vi "Calculate_Velocity.vi"(2 "Times":T1 {"Accel fractional distance" format="%.2f"; "Accel time" format="%.7f"; "Total travel time" format="%.7f"}, 5 "Revs to travel":dbl format="%.2f") -> (0 "Acceleration":dbl format="%.2f", 1 "Max Velocity":dbl format="%.2f")   [LabVIEW 2018]
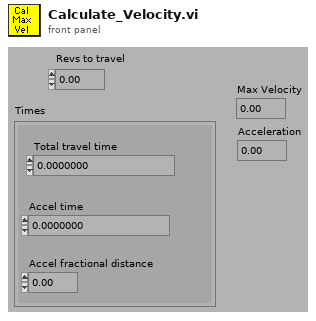
[diagram p1: front panel]
types:
  T1 = cluster{"Total travel time":dbl, "Accel time":dbl, "Accel fractional distance":dbl}
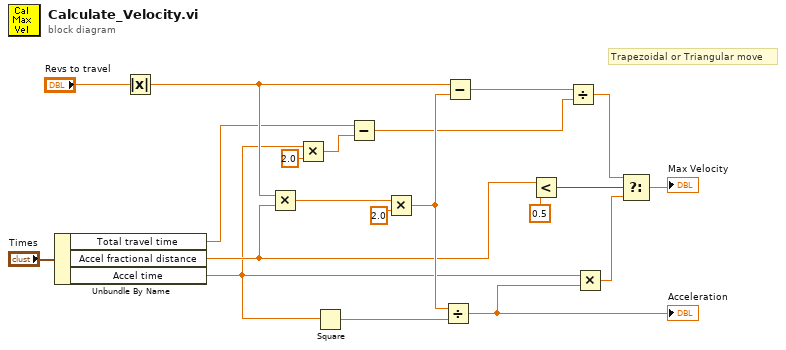
[diagram p0: block diagram]
diagram:
  # "Trapezoidal or Triangular move"
  n1 = Unbundle By Name("Times") -> ("Total travel time"=w1:dbl, "Accel fractional distance"=w3:dbl, "Accel time"=w2:dbl)
  n2 = Absolute Value(x="Revs to travel") -> (abs(x)=w14:dbl)
  n3 = Multiply(x=w14, y=w3) -> (x*y=w19:dbl)
  n4 = Multiply(x=w2, y=2.0) -> (x*y=w15:dbl)
  n5 = Square(x=w2) -> (x^2=w17:dbl)
  n6 = Subtract(x=w1, y=w15) -> (x-y=w11:dbl)
  n7 = Multiply(x=w19, y=2.0) -> (x*y=w13:dbl)
  n8 = Divide(x=w13, y=w17) -> (x/y=w6:dbl)
  "Acceleration" <- w6
  n9 = Subtract(x=w14, y=w13) -> (x-y=w12:dbl)
  n10 = Less?(x=w3, y=0.5) -> (x < y?=w9:bool)
  n11 = Divide(x=w12, y=w11) -> (x/y=w8:dbl)
  n12 = Multiply(x=w2, y=w6) -> (x*y=w5:dbl)
  n13 = Select(t=w8, s=w9, f=w5) -> (s? t:f=→"Max Velocity":dbl)
